vi "Get Question.vi"(0 "Candidate ID":string, 5 "Question_ID":string, 11 "error in (no error)":errorcluster) -> (4 "Test Description":T1, 15 "error out":errorcluster)   [LabVIEW 2014, in "Coding Platform.lvlib"]
uses:
  Coding Platform.lvlib
  Typedefs/User Event Operations.ctl
  Datatypes/Get Question.ctl
  Datatypes/Question Response.ctl
  Datatypes/Test Description.ctl
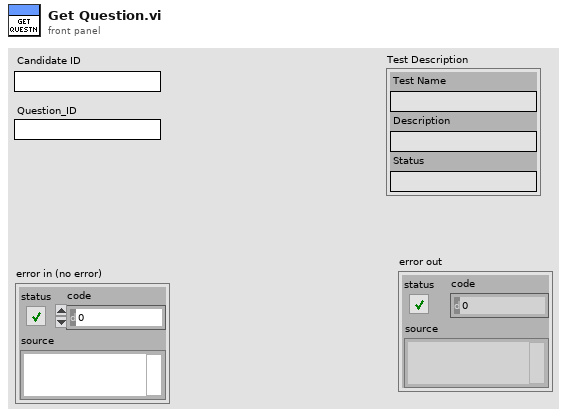
[diagram p1: front panel]
types:
  T1 = typedef "Coding Platform.lvlib/Test Description.ctl" = cluster{"Test Name":string, "Description":string, "Status":string}
  T2 = typedef "Coding Platform.lvlib/Get Question.ctl" = cluster{"CandidateID":string, "Question_ID":string, "notifier":refnum<notifier>}
  T3 = typedef "Coding Platform.lvlib/Question Response.ctl" = cluster{"Question Title":string, "Question":string, "Description":string}
  T4 = typedef "Coding Platform.lvlib/User Event Operations.ctl" = enum16{"Create", "Genereate", "Destroy", "Get Reference"}
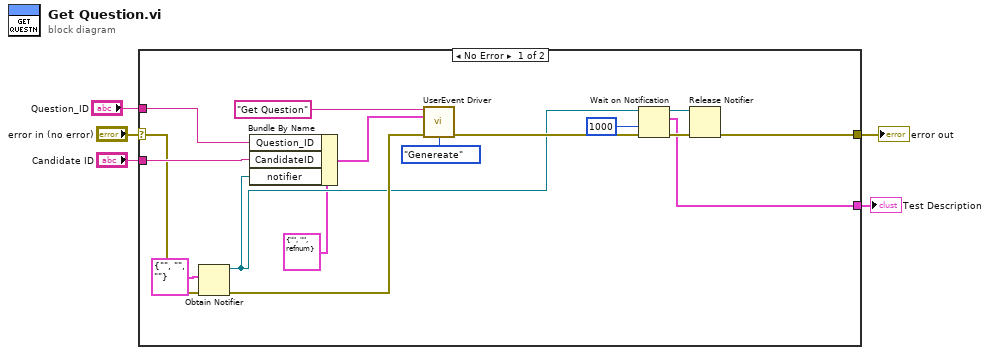
[diagram p0: block diagram]
diagram:
  n1 = case shown="No Error" "error in (no error)" {
    selector: "error in (no error)" -> [w10 w22]
    tunnel: [w14 w22] -> w5
    tunnel: "Candidate ID" -> [w17 _]
    tunnel: [w12 _] -> w2
    tunnel: "Question_ID" -> [w6 _]
    frame No Error {
      n2 = Obtain Notifier(notification data type=T3 {"Question Title"="", "Question"="", "Description"=""}, error in (no error)=w10) -> (notifier out=w8:refnum<notifier>, error out=w11:errorcluster)  [unwired: 2 in, 1 out]
      n3 = Bundle By Name(cluster=T2 {"CandidateID"="", "Question_ID"="", "notifier"=refnum} ("Get Question"), "Question_ID"=w6, "CandidateID"=w17, "notifier"=w8) -> (w18:T2)
      n4 = call "UserEvent Driver.vi"("Message"="Get Question", "Data"=w18, "error in (no error)"=w11, "Operations(Get Reference)"=User_Event_Operations."Genereate") -> ("error out"=w21:errorcluster)  [unwired: 10 in, 1 out]
      n5 = Wait on Notification(notifier=w8, timeout in ms (-1)=1000, error in (no error)=w21) -> (notifier out=w13:refnum<notifier>, notification=w12:T3, error out=w16:errorcluster)  [unwired: 1 in, 1 out]
      n6 = Release Notifier(notifier=w13, error in (no error)=w16) -> (error out=w14:errorcluster)  [unwired: 1 in, 2 out]
    }
    frame Error {
    }
  }
  "error out" <- w5
  "Test Description" <- w2
